vi "Drive_Test.vi"(11 "Joystick_In":T1) -> ()   [LabVIEW 2019]
uses:
  Utility_VIs/Joystick_Controls.ctl
  Subsystems/Drive/Drive_Cluster.ctl
  Subsystems/Drive/Drive_States.ctl
  Globals/Drive_Globals.vi
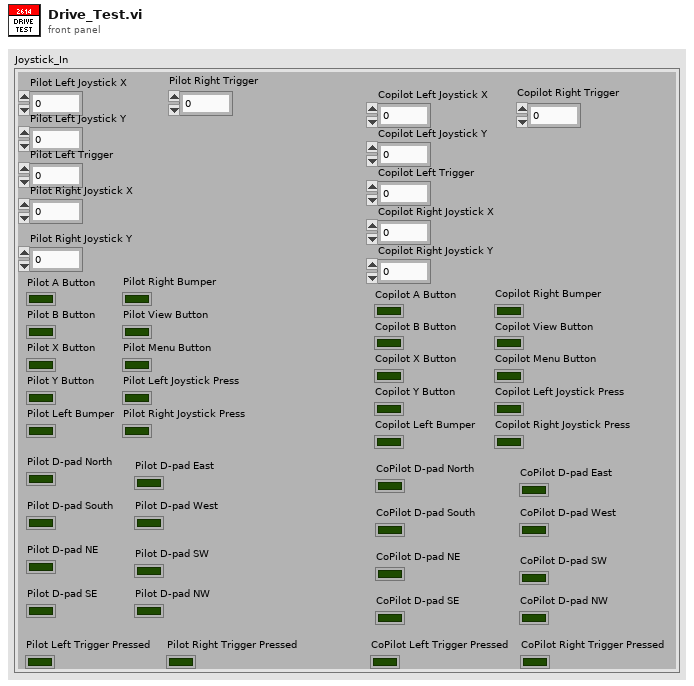
[diagram p1: front panel]
types:
  T1 = typedef "Joystick_Controls.ctl" = cluster{"Pilot Left Joystick X":dbl, "Pilot Left Joystick Y":dbl, "Pilot A Button":bool, "Pilot B Button":bool, "Pilot X Button":bool, "Pilot Y Button":bool, "Pilot Left Bumper":bool, "Pilot Right Bumper":bool, "Pilot View Button":bool, "Pilot Menu Button":bool, "Pilot Left Joystick Press":bool, "Pilot Right Joystick Press":bool, "Pilot Left Trigger":dbl, "Pilot Right Joystick X":dbl, "Pilot Right Joystick Y":dbl, "Pilot Right Trigger":dbl, "Copilot Left Joystick X":dbl, "Copilot Left Joystick Y":dbl, "Copilot A Button":bool, "Copilot B Button":bool, "Copilot X Button":bool, "Copilot Y Button":bool, "Copilot Left Bumper":bool, "Copilot Right Bumper":bool, "Copilot View Button":bool, "Copilot Menu Button":bool, "Copilot Left Joystick Press":bool, "Copilot Right Joystick Press":bool, "Copilot Left Trigger":dbl, "Copilot Right Joystick X":dbl, "Copilot Right Joystick Y":dbl, "Copilot Right Trigger":dbl, "Pilot D-pad North":bool, "Pilot D-pad South":bool, "Pilot D-pad East":bool, "Pilot D-pad West":bool, "Pilot D-pad NE ":bool, "Pilot D-pad SE":bool, "Pilot D-pad SW":bool, "Pilot D-pad NW":bool, "CoPilot D-pad North":bool, "CoPilot D-pad South":bool, "CoPilot D-pad East":bool, "CoPilot D-pad West":bool, "CoPilot D-pad NE":bool, "CoPilot D-pad SE":bool, "CoPilot D-pad SW":bool, "CoPilot D-pad NW":bool, "Pilot Left Trigger Pressed":bool, "Pilot Right Trigger Pressed":bool, "CoPilot Left Trigger Pressed":bool, "CoPilot Right Trigger Pressed":bool}
  T2 = typedef "Drive_Cluster.ctl" = cluster{"Control_State":T3, "Angular_Throttle":dbl, "Linear_Throttle":dbl, "Torque_Changing":bool}
  T3 = typedef "Drive_States.ctl" = enum16{"Percent_Voltage_Control", "Speed_Control"}
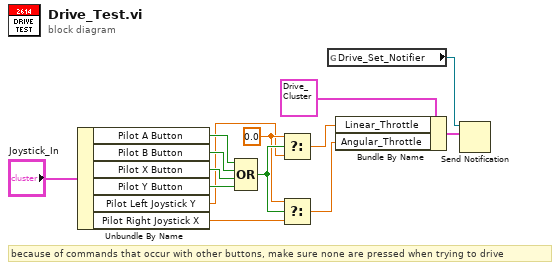
[diagram p0: block diagram]
diagram:
  w4 = 0.0 ("t")
  # "because of commands that occur with other buttons, make sure none are pressed when trying to drive"
  n1 = Unbundle By Name("Joystick_In") -> ("Pilot A Button"=w10:bool, "Pilot B Button"=w9:bool, "Pilot X Button"=w8:bool, "Pilot Y Button"=w7:bool, "Pilot Left Joystick Y"=w2:dbl, "Pilot Right Joystick X"=w3:dbl)
  n2 = Compound Arithmetic op=OR(w10, w9, w8, w7) -> (w5:bool)
  n3 = Select(t=w4, s=w5, f=w2) -> (s? t:f=w1:dbl)
  n4 = Select(t=w4, s=w5, f=w3) -> (s? t:f=w6:dbl)
  n5 = global read "Drive_Globals.vi" "Drive_Set_Notifier"() -> (w14:refnum<notifier>)
  n6 = Bundle By Name(cluster=T2 {"Control_State"=enum."Percent_Voltage_Control", "Angular_Throttle"=0.0, "Linear_Throttle"=0.0, "Torque_Changing"=FALSE} ("notification"), "Linear_Throttle"=w1, "Angular_Throttle"=w6) -> (w12:T2)
  n7 = Send Notification(notification=w12, notifier=w14) -> ()  [unwired: 1 in, 2 out]
